vi "File Check.vi"(0 "AKLH Filenames":string[](array[string]), 1 "Data Log Dirs":path[](array[path]), 2 "AKLH Today Dirs":path[](array[path]), 3 "File Check Time (ms) In":u32, 4 "File Check Period (ms)":u32, 5 "FC Data Log Times In":u32[](array[numeric]), 6 "Data Log Times IN":u32[](array[numeric]), 7 "FC AKLH Log Times In":u32[][](array[numeric]), 8 "AKLH Log Times IN":u32[][](array[numeric]), 9 "Data Log Sizes In":i64[](array[numeric]), 11 "AKLH Log Sizes In":i64[][](array[numeric])) -> (14 "File Check Time (ms) Out":u32, 15 "FC Data Log Times Out":u32[](array[numeric]), 16 "FC AKLH Log Times Out":u32[][](array[numeric]), 17 "Data Log Sizes Out":i64[](array[numeric]), 18 "AKLH Log Sizes Out":i64[][](array[numeric]))   [LabVIEW 2019]
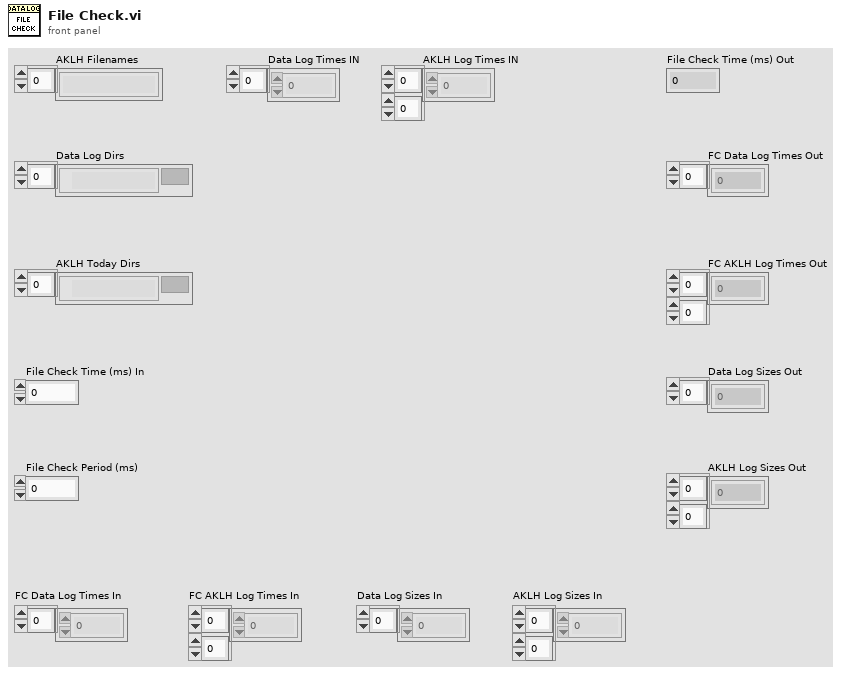
[diagram p1: front panel]
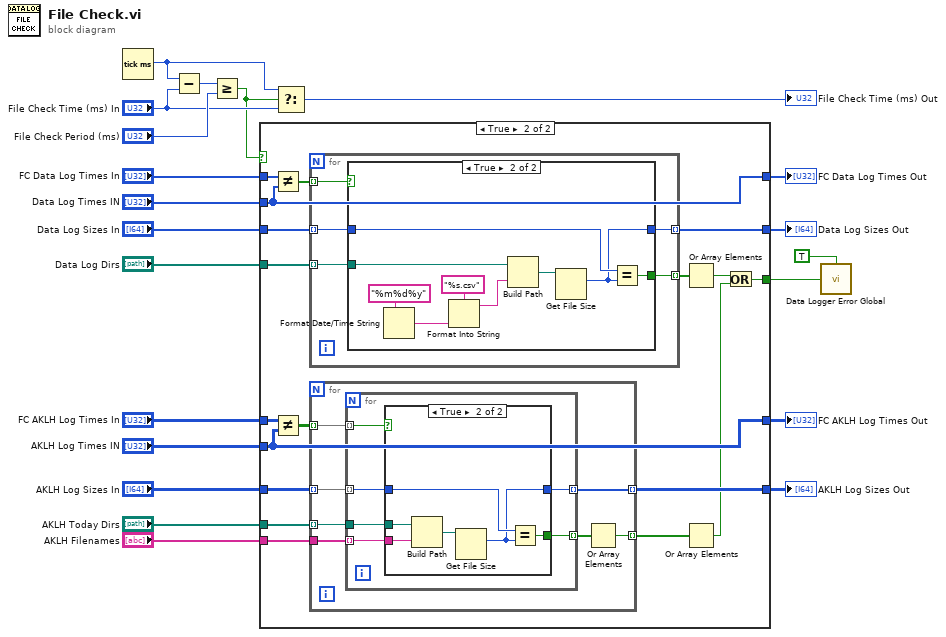
[diagram p0: block diagram]
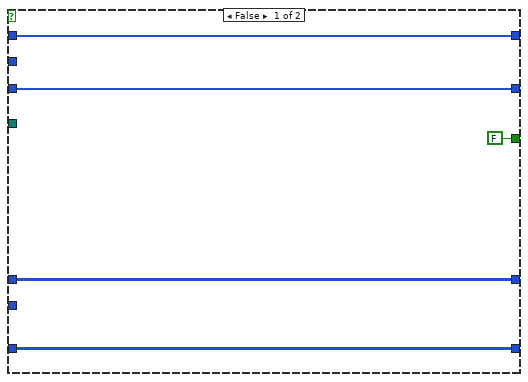
[diagram p2: hidden frame]
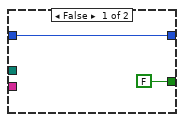
[diagram p3: hidden frame]
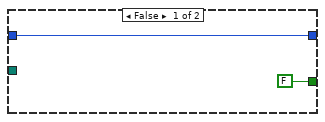
[diagram p4: hidden frame]
diagram:
  n1 = Tick Count (ms)() -> (millisecond timer value=w19:u32)
  n2 = Subtract(x=w19, y="File Check Time (ms) In") -> (x-y=w21:u32)
  n3 = Greater Or Equal?(x=w21, y="File Check Period (ms)") -> (x >= y?=w16:bool)
  n4 = case shown="True" w16 {
    tunnel: "FC Data Log Times In" -> [w26 w44]
    tunnel: "FC AKLH Log Times In" -> [w25 w43]
    tunnel: [w26 w41] -> w13
    tunnel: [w25 w42] -> w12
    tunnel: "Data Log Times IN" -> [_ w41]
    tunnel: "AKLH Log Times IN" -> [_ w42]
    tunnel: "Data Log Sizes In" -> [w24 w38]
    tunnel: [w24 w37] -> w8
    tunnel: "AKLH Log Sizes In" -> [w23 w35]
    tunnel: [w23 w32] -> w6
    tunnel: "Data Log Dirs" -> [_ w39]
    tunnel: "AKLH Today Dirs" -> [_ w34]
    tunnel: "AKLH Filenames" -> [_ w33]
    tunnel: [FALSE w27] -> w2
    frame False {
    }
    frame True {
      n5 = Not Equal?(x=w44, y=w41) -> (x != y?=w40:bool[])
      n6 = Not Equal?(x=w43, y=w42) -> (x != y?=w36:bool[][])
      n7 = for {
        tunnel: w40 -> [w70] mode=indexing
        tunnel: w39 -> [w67] mode=indexing
        tunnel: w38 -> [w69] mode=indexing
        tunnel: [w68] -> w37 mode=indexing
        tunnel: [w66] -> w30 mode=indexing
        n8 = case shown="True" w70 {
          tunnel: w69 -> [w72 w81]
          tunnel: [w72 w80] -> w68
          tunnel: w67 -> [_ w74]
          tunnel: [FALSE w79] -> w66
          frame False {
          }
          frame True {
            n9 = Format Date/Time String(time format string (%c)="%m%d%y") -> (date/time string=w77:string)  [unwired: 2 in]
            n10 = Format Into String(format string="%s.csv", w77) -> (resulting string=w75:string)  [unwired: 2 in, 1 out]
            n11 = Build Path(base path=w74, name or relative path=w75) -> (appended path=w73:path)
            n12 = Get File Size(file=w73) -> (size (in bytes)=w80:i64)  [unwired: 1 in, 2 out]
            n13 = Equal?(x=w81, y=w80) -> (x = y?=w79:bool)
          }
        }
      }
      n14 = for {
        tunnel: w36 -> [w51] mode=indexing
        tunnel: w34 -> [w48] mode=indexing
        tunnel: w35 -> [w50] mode=indexing
        tunnel: [w49] -> w32 mode=indexing
        tunnel: w33 -> [w47]
        tunnel: [w45] -> w31 mode=indexing
        n15 = for {
          tunnel: w51 -> [w57] mode=indexing
          tunnel: w50 -> [w56] mode=indexing
          tunnel: [w55] -> w49 mode=indexing
          tunnel: w48 -> [w54]
          tunnel: [w53] -> w46 mode=indexing
          tunnel: w47 -> [w52] mode=indexing
          n16 = case shown="True" w57 {
            tunnel: w56 -> [w59 w65]
            tunnel: [w59 w64] -> w55
            tunnel: w54 -> [_ w62]
            tunnel: [FALSE w63] -> w53
            tunnel: w52 -> [_ w60]
            frame False {
            }
            frame True {
              n17 = Build Path(base path=w62, name or relative path=w60) -> (appended path=w61:path)
              n18 = Get File Size(file=w61) -> (size (in bytes)=w64:i64)  [unwired: 1 in, 2 out]
              n19 = Equal?(x=w65, y=w64) -> (x = y?=w63:bool)
            }
          }
        }
        n20 = Or Array Elements(Boolean array=w46) -> (logical OR=w45:bool)
      }
      n21 = Or Array Elements(Boolean array=w30) -> (logical OR=w29:bool)
      n22 = Or Array Elements(Boolean array=w31) -> (logical OR=w28:bool)
      n23 = Or(x=w29, y=w28) -> (x .or. y?=w27:bool)
    }
  }
  "FC Data Log Times Out" <- w13
  "FC AKLH Log Times Out" <- w12
  "Data Log Sizes Out" <- w8
  "AKLH Log Sizes Out" <- w6
  n24 = Select(t=w19, s=w16, f="File Check Time (ms) In") -> (s? t:f=→"File Check Time (ms) Out":u32)
  n25 = call "Data Logger Error Global.vi"("Write (F)"=TRUE, "Datalog Error In"=w2) -> ()  [unwired: 13 in, 1 out]
